vi "Init.vi"(0 "IV in":refnum<class "IV.lvclass">, 5 "Path":path=path "C:/Users/Sergei/Documents", 7 "Measurement2D.lvclass":refnum<class "Measurement2D.lvclass">, 9 "Data2D.lvclass":refnum<class "Data2D.lvclass">, 11 "error in (no error)":errorcluster) -> (4 "IV out":refnum<class "IV.lvclass">, 15 "error out":errorcluster)   [LabVIEW 2018, in "IV.lvclass"]
uses:
  IV.lvclass
  Abstract/Measurement/Measurement2D/Measurement2D.lvclass
  Abstract/Data/Data2D/Data2D.lvclass
  Abstract/Experiment/Experiment2D/Experiment2D.lvclass
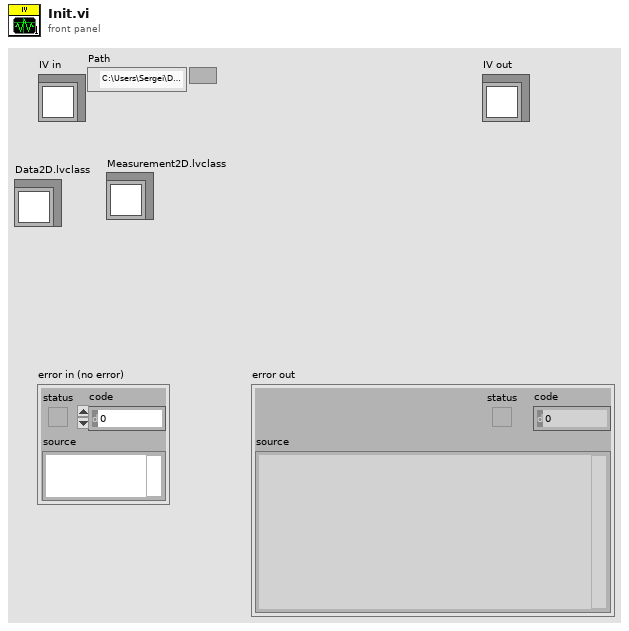
[diagram p1: front panel]
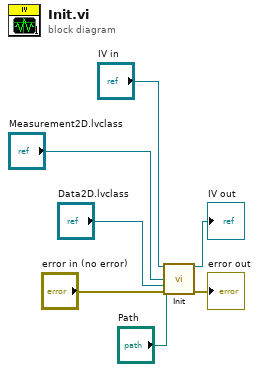
[diagram p0: block diagram]
diagram:
  n1 = call-parent "Init.vi"("Experiment2D in"="IV in", "Path"="Path", "Measurement2D.lvclass"="Measurement2D.lvclass", "Data2D.lvclass"="Data2D.lvclass", "error in (no error)"="error in (no error)") -> ("Experiment2D out"=→"IV out":refnum<class "IV.lvclass">, "error out"=→"error out":errorcluster)  [unwired: 9 in]
